vi "New Verify Combinations.vi"   [LabVIEW 2020, in "Caraya.Extension.lvlib"]
uses:
  Caraya.Extension.lvlib
  <vilib>/addons/_JKI Toolkits/Caraya/classes/Test/Test.lvclass
  bacf86de-937c-4a87-a907-1b0971078436.vi
  1b635337-1e38-4d08-aae1-8dabe6c40bc9.vi
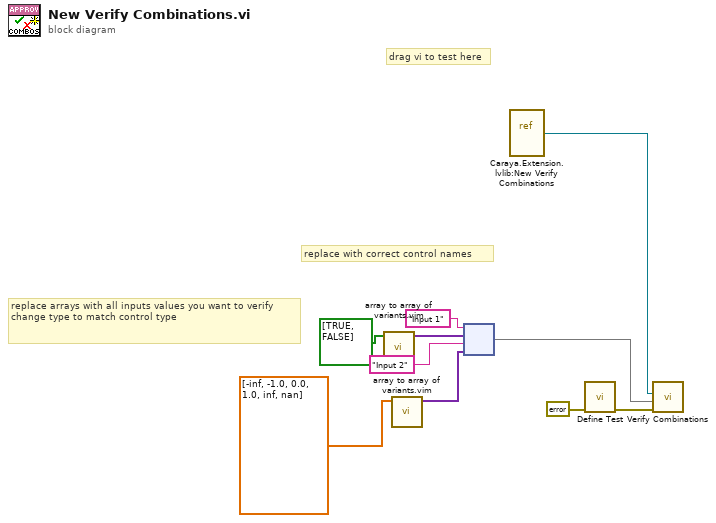
[diagram p0: block diagram]
diagram:
  # "replace arrays with all inputs values you want to verify\nchange type to match control type"
  # "replace with correct control names"
  # "drag vi to test here"
  n1 = call "array to array of variants.vim"("Array in"=bool[] [TRUE, FALSE]) -> ("Array out"=w4:variant[])  [unwired: 10 in]
  n2 = call "array to array of variants.vim"("Array in"=dbl[] [-inf, -1.0, 0.0, 1.0, inf, nan]) -> ("Array out"=w3:variant[])  [unwired: 10 in]
  n3 = node ("Build Map")("Input 1" ("key"), w4, "Input 2" ("key"), w3) -> (w1:map{string, variant[]})
  n4 = vi-ref "Caraya.Extension.lvlib:New Verify Combinations.vi"() -> (w8:refnum<vi>)
  n5 = call <vilib>:"Define Test.vi"("error in (no error)"=errorcluster {"status"=FALSE, "code"=0, "source"=""}) -> ("error out"=w9:errorcluster)  [unwired: 9 in, 1 out]
  n6 = call "Verify Combinations.vi"("error in"=w9, "ctl label -> value var[]"=w1, "VI Refnum"=w8) -> ()  [unwired: 7 in, 2 out]
